vi "SetUSB5AoDataFifo.vi"(8 "错误输入（无错误）":errorcluster, 9 "Voltage":sgl[](array[numeric]), 10 "Chan":u8, 11 "DevIndex":i32) -> (0 "错误输出":errorcluster, 3 "DevIndex Out":i32)   [LabVIEW 2020]
uses:
  lib/x64/USB5000.dll
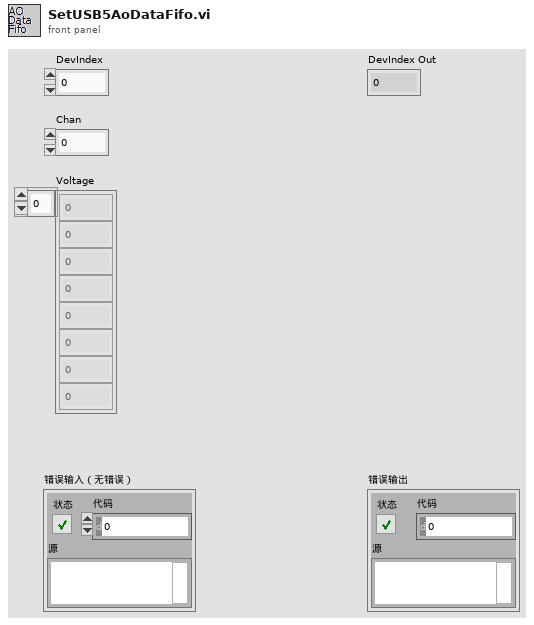
[diagram p1: front panel]
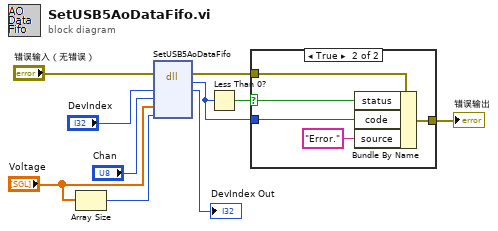
[diagram p0: block diagram]
diagram:
  n1 = Array Size(array="Voltage") -> (size(s)=w5:i32)
  n2 = dll-call lib="C:/Users/phosense/Downloads/USB-5000/USB-5000_LabVIEW/lib/x64/USB5000.dll" fn="SetUSB5AoDataFifo"(error in="错误输入（无错误）", "DevIndex"="DevIndex", "Chan"="Chan", "Voltage"="Voltage", "Len"=w5) -> (error out=w3:errorcluster, "返回类型"=w2:i32, "DevIndex"=→"DevIndex Out":i32)  [unwired: 5 in, 1 out]
  n3 = Less Than 0?(x=w2) -> (x < 0?=w4:bool)
  n4 = case shown="True" w4 {
    selector: w4 -> [_ w12]
    tunnel: [w11 w14] -> w1
    tunnel: w2 -> [_ w16]
    tunnel: w3 -> [w11 w13]
    frame False {
    }
    frame True {
      n5 = Bundle By Name(cluster=w13, "status"=w12, "code"=w16, "source"="Error." ("error message (\"\")")) -> (w14:errorcluster)
    }
  }
  "错误输出" <- w1
